vi "Read Access Index.vi"(8 "error in (no error)":errorcluster, 11 "Var_Index in":refnum<class "Var_Index.lvclass">) -> (0 "error out":errorcluster, 2 "Access Index":u32, 3 "Var_Index out":refnum<class "Var_Index.lvclass">)   [LabVIEW 2021, in "Var_Index.lvclass"]
uses:
  Var_Index.lvclass
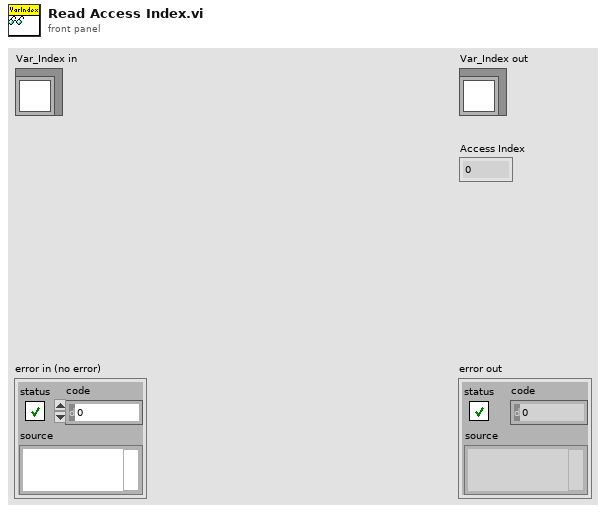
[diagram p1: front panel]
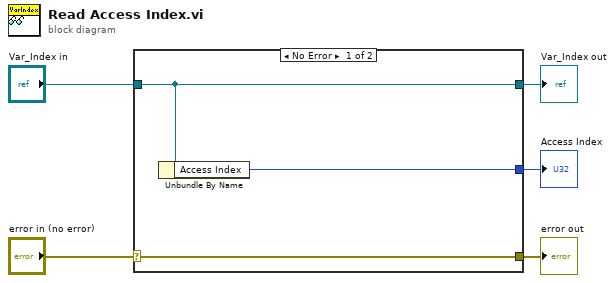
[diagram p0: block diagram]
diagram:
  n1 = case shown="No Error" "error in (no error)" {
    selector: "error in (no error)" -> [w8 w9]
    tunnel: [w8 w9] -> w4
    tunnel: [w7 w10] -> w2
    tunnel: "Var_Index in" -> [w7 w10]
    tunnel: [w6 _] -> w1
    frame No Error {
      n2 = Unbundle By Name(w7) -> ("Access Index"=w6:u32)
    }
    frame Error {
    }
  }
  "error out" <- w4
  "Var_Index out" <- w2
  "Access Index" <- w1
